vi "Stop Core.vi"(10 "final error code":i32, 11 "Monitored Actor in":refnum<class "Monitored Actor.lvclass">) -> (3 "Monitored Actor out":refnum<class "Monitored Actor.lvclass">)   [LabVIEW 2018, in "Monitored Actor.lvlib" / "Monitored Actor.lvclass"]
doc: "In addition to the following, this method also sends a message to the monitor to notify it that the actor has stopped execution.\n\n(<B>Filename</B>: Actor Framework.lvlib:Actor.lvclass:Stop Core.vi)\n\nDefines what the actor does before it stops. Use the <B>final error code</B> input to determine whether the actor shut down in response to an error.\n\nBy default, this method does nothing. A descendant class may override it to define behavior, such as shutting down any processes the actor initiated in its override of the Actor Core method.\n\nCopyright: MGI\nAuthored by: Derek Trepanier"
uses:
  Monitored Actor.lvclass
  Monitored Actor.lvclass/Monitored Actor.ctl
  Actor Monitor/Actor Monitor Messages/Actor Stopped Msg/Actor Stopped Msg.lvclass/Actor Stopped Msg.ctl
  <vilib>/ActorFramework/Message Enqueuer/Message Enqueuer.lvclass/Message Enqueuer.ctl
  <vilib>/ActorFramework/Message Enqueuer/Enqueue.vi
  Actor Monitor/Actor Monitor Messages/Actor Stopped Msg/Actor Stopped Msg.lvclass
  C:/Program Files (x86)/National Instruments/LabVIEW 2018/vi.lib/ActorFramework/Message/Message.lvclass
  <vilib>/ActorFramework/Message Priority Queue/Priority Enqueue.vi
  <vilib>/ActorFramework/Actor/Actor.lvclass
  Actor Monitor/Actor/Actor Monitor.lvclass
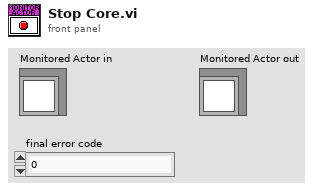
[diagram p1: front panel]
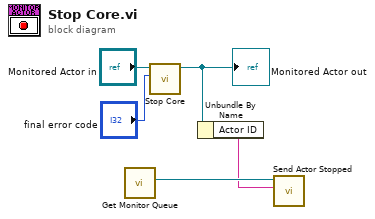
[diagram p0: block diagram]
diagram:
  n1 = call "Get Monitor Queue.vi"() -> ("Caller Enqueuer"=w3:refnum<class "Message Enqueuer.lvclass">)  [unwired: 11 in]
  n2 = call-parent "Stop Core.vi"("final error code"="final error code", "Actor in"="Monitored Actor in") -> ("Actor out"=w2:refnum<class "Monitored Actor.lvclass">)  [unwired: 9 in]
  "Monitored Actor out" <- w2
  n3 = Unbundle By Name(w2) -> ("Actor ID"=w1:string)
  n4 = call "Send Actor Stopped.vi"("Actor Core Name"=w1, "Message Enqueuer"=w3) -> ()  [unwired: 8 in, 2 out]
